vi "SaveDataScalerV830.vi"(6 "Module":string="QDC Data", 8 "error in (no error)":errorcluster, 9 "Buff":u32[](array[numeric]), 10 "File Handle":T1 format="%.0x", 11 "Group Name":string) -> (0 "error out":errorcluster)   [LabVIEW 2014]
uses:
  <vilib>/addons/h5labview2/base/hid_t.ctl
  <vilib>/addons/h5labview2/base/lib_path.vi
  <vilib>/addons/h5labview2/base/H5Equery.vi
  <vilib>/addons/h5labview2/dataset/H5Dwrite.llb/H5Dwrite.xnode
  <vilib>/addons/h5labview2/group/H5G.lvlib
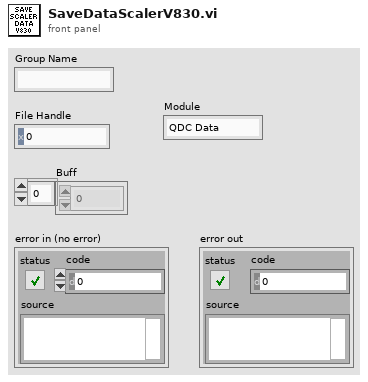
[diagram p1: front panel]
types:
  T1 = typedef "hid_t.ctl" = i32
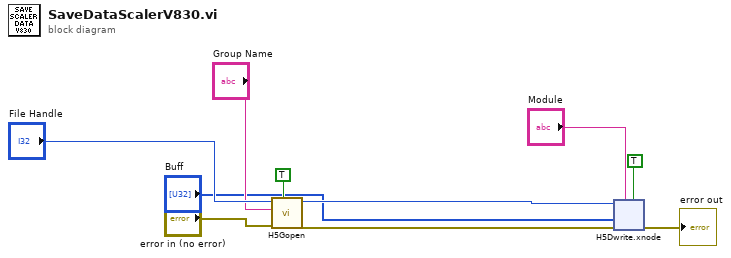
[diagram p0: block diagram]
diagram:
  n1 = call <vilib>:"H5Gopen.vi"("create? (F)"=TRUE, "error in (no error)"="error in (no error)", "name"="Group Name", "ref in"="File Handle") -> ("error out"=w2:errorcluster, "group out"=w8:T1)  [unwired: 6 in]
  n2 = xnode "H5Dwrite.xnode"("replace? (F)"=TRUE, "dataset name"="Module", "error in (no error)"=w2, "data"="Buff", "ref in"=w8) -> ("error out"=→"error out":errorcluster)  [unwired: 2 in, 2 out]
